vi "Write Numeric Char.vi"(8 "error in (no error)":errorcluster, 10 "Numeric In":string, 11 "HT16K33 LED Driver  in":refnum<class "HT16K33 LED Driver.lvclass">) -> (0 "error out":errorcluster, 3 "HT16K33 LED Driver out":refnum<class "HT16K33 LED Driver.lvclass">)   [LabVIEW 2020, in "CTI-Peripheral.lvlib" / "HT16K33 LED Driver.lvclass"]
uses:
  HT16K33 LED Driver.lvclass
  HT16K33 LED Driver.lvclass/HT16K33 LED Driver.ctl
  CTI/I2C Connection/I2C Connection.lvclass/I2C Connection.ctl
  CTI/Session/I2C Write Data.vi
  CTI/I2C Connection/I2C Connection.lvclass
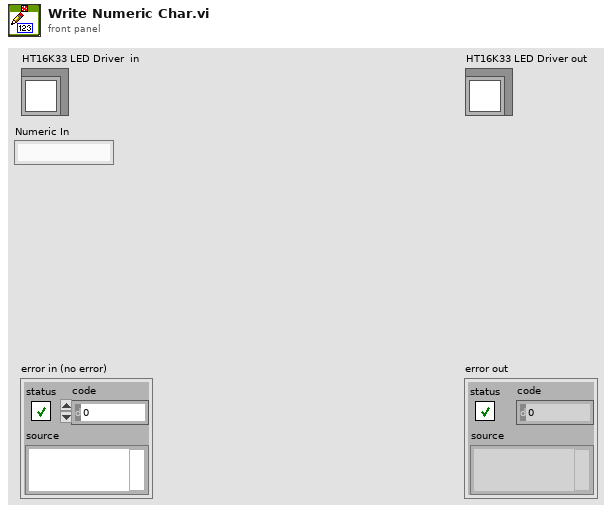
[diagram p1: front panel]
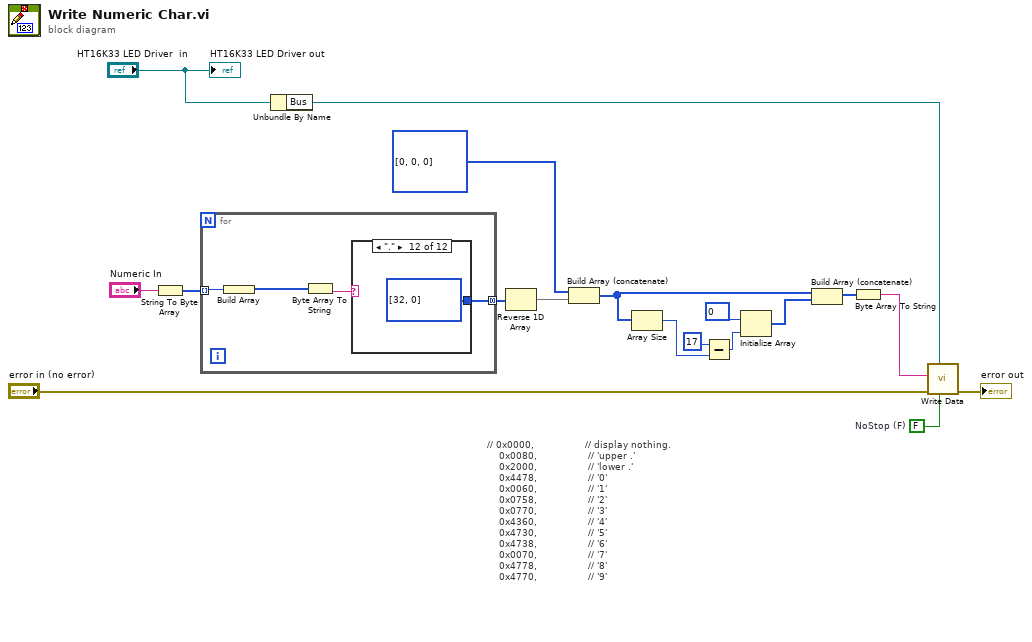
[diagram p0: block diagram]
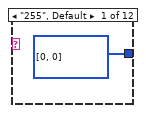
[diagram p2: hidden frame]
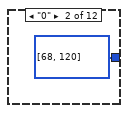
[diagram p3: hidden frame]
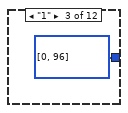
[diagram p4: hidden frame]
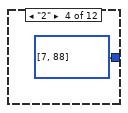
[diagram p5: hidden frame]
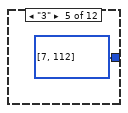
[diagram p6: hidden frame]
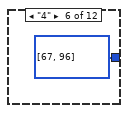
[diagram p7: hidden frame]
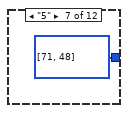
[diagram p8: hidden frame]
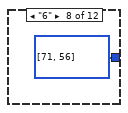
[diagram p9: hidden frame]
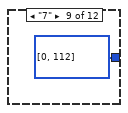
[diagram p10: hidden frame]
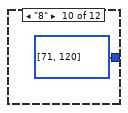
[diagram p11: hidden frame]
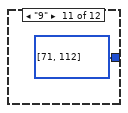
[diagram p12: hidden frame]
diagram:
  w18 = FALSE  # NoStop (F)
  # "// 0x0000,                 // display nothing.\n    0x0080,                 // 'upper .'\n    0x2000,                 // 'lower .'\n    0x4478,                 // '0'\n    0x0060,                 // '1'\n    0x0758,                 // '2'\n    0x0770,                 // '3'\n    0x4360,                 // '4'\n    0x4730,                 // '5'\n    0x4738,                 // '6'\n    0x0070,                 // '7'\n    0x4778,                 // '8'\n    0x4770,                 // '9'"
  n1 = String To Byte Array(string="Numeric In") -> (unsigned byte array=w13:u8[])
  n2 = for {
    tunnel: w13 -> [w21] mode=indexing
    tunnel: [w19] -> w10 mode=concatenating
    n3 = Build Array(w21) -> (w20:u8[])
    n4 = Byte Array To String(unsigned byte array=w20) -> (string=w22:string)
    n5 = case shown="\".\"" w22 {
      tunnel: [u8[] [0, 0] u8[] [68, 120] u8[] [0, 96] u8[] [7, 88] u8[] [7, 112] u8[] [67, 96] u8[] [71, 48] u8[] [71, 56] u8[] [0, 112] u8[] [71, 120] u8[] [71, 112] u8[] [32, 0]] -> w19
      frame "255", Default {
      }
      frame "0" {
      }
      frame "1" {
      }
      frame "2" {
      }
      frame "3" {
      }
      frame "4" {
      }
      frame "5" {
      }
      frame "6" {
      }
      frame "7" {
      }
      frame "8" {
      }
      frame "9" {
      }
      frame "." {
      }
    }
  }
  n6 = Unbundle By Name("HT16K33 LED Driver  in") -> ("Bus"=w14:refnum<class "I2C Connection.lvclass">)
  n7 = Reverse 1D Array(array=w10) -> (reversed array=w1:u8[])
  n8 = Build Array (concatenate)(u8[] [0, 0, 0], w1) -> (w5:u8[])
  n9 = Array Size(array=w5) -> (size(s)=w7:i32)
  n10 = Subtract(x=17, y=w7) -> (x-y=w3:i32)
  n11 = Initialize Array(u8 0, w3) -> (w2:u8[])
  n12 = Build Array (concatenate)(w5, w2) -> (w6:u8[])
  n13 = Byte Array To String(unsigned byte array=w6) -> (string=w11:string)
  n14 = call "Write Data.vi"("NoStop (F)"=w18, "I2C Connection"=w14, "error in (no error)"="error in (no error)", "Data"=w11) -> ("error out"=→"error out":errorcluster)  [unwired: 7 in]
  "HT16K33 LED Driver out" <- "HT16K33 LED Driver  in"
